vi "Create New Assert.vi"(6 "Variant in":variant, 7 "Shift Pressed?":bool, 8 "error in (no error)":errorcluster, 10 "QD Combo Box Ref":refnum<vi>, 11 "QD Launch VI Ref":refnum<vi>) -> (0 "error out":errorcluster, 4 "Variant out":variant)   [LabVIEW 2016]
doc: "Allows the user to define and insert a new assert statement onto a wire - supports I32, Double, String and Boolean data types currently\n\nDefault Shortcut - S"
panel:
  in  "Undo Name":string="Quick Drop Keyboard Shortcut"
  # "Do not change the connector pane of this VI.\n\nSee the block diagram for directions on how to use this template."
  # "Specify the name of the Undo transaction"
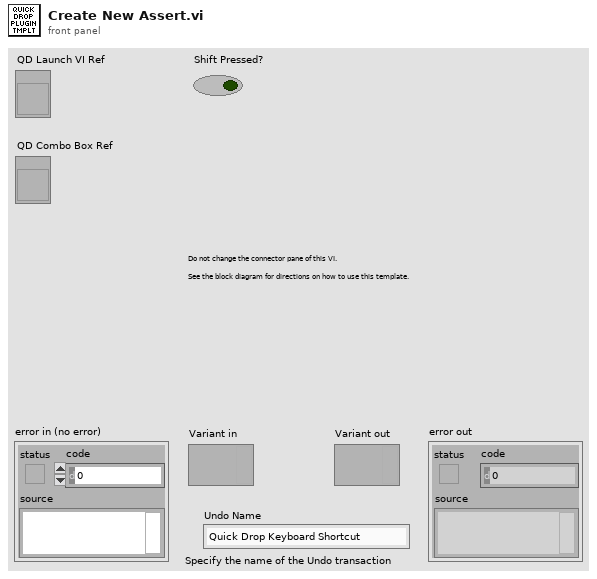
[diagram p1: front panel]
types:
  T1 = typedef "NI_Data Type.lvlib/Data Type.ctl" = enum8{"Invalid Type", "Void", "I8", "I16", "I32", "I64", "U8", "U16", "U32", "U64", "Single Float", "Double Float", "Extended Float", "Single Complex", "Double Complex", "Extended Complex", "Enum U8", "Enum U16", "Enum U32", "Enum U64", "Single Float With Unit", "Double Float With Unit", "Extended Float With Unit", "Single Complex with Unit", "Double Complex with Unit", "Extended Complex with Unit", "Boolean", "String", "Path", "Picture", "Tag", "Array", "Cluster", "Variant", "LV Variant", "Waveform", "Timestamp", "Digital Waveform", "Digital Data", "ExpressData", "Refnum", "External Data", "VI", "Poly VI", "LabVIEW Class Instance", "Fixed Point"}
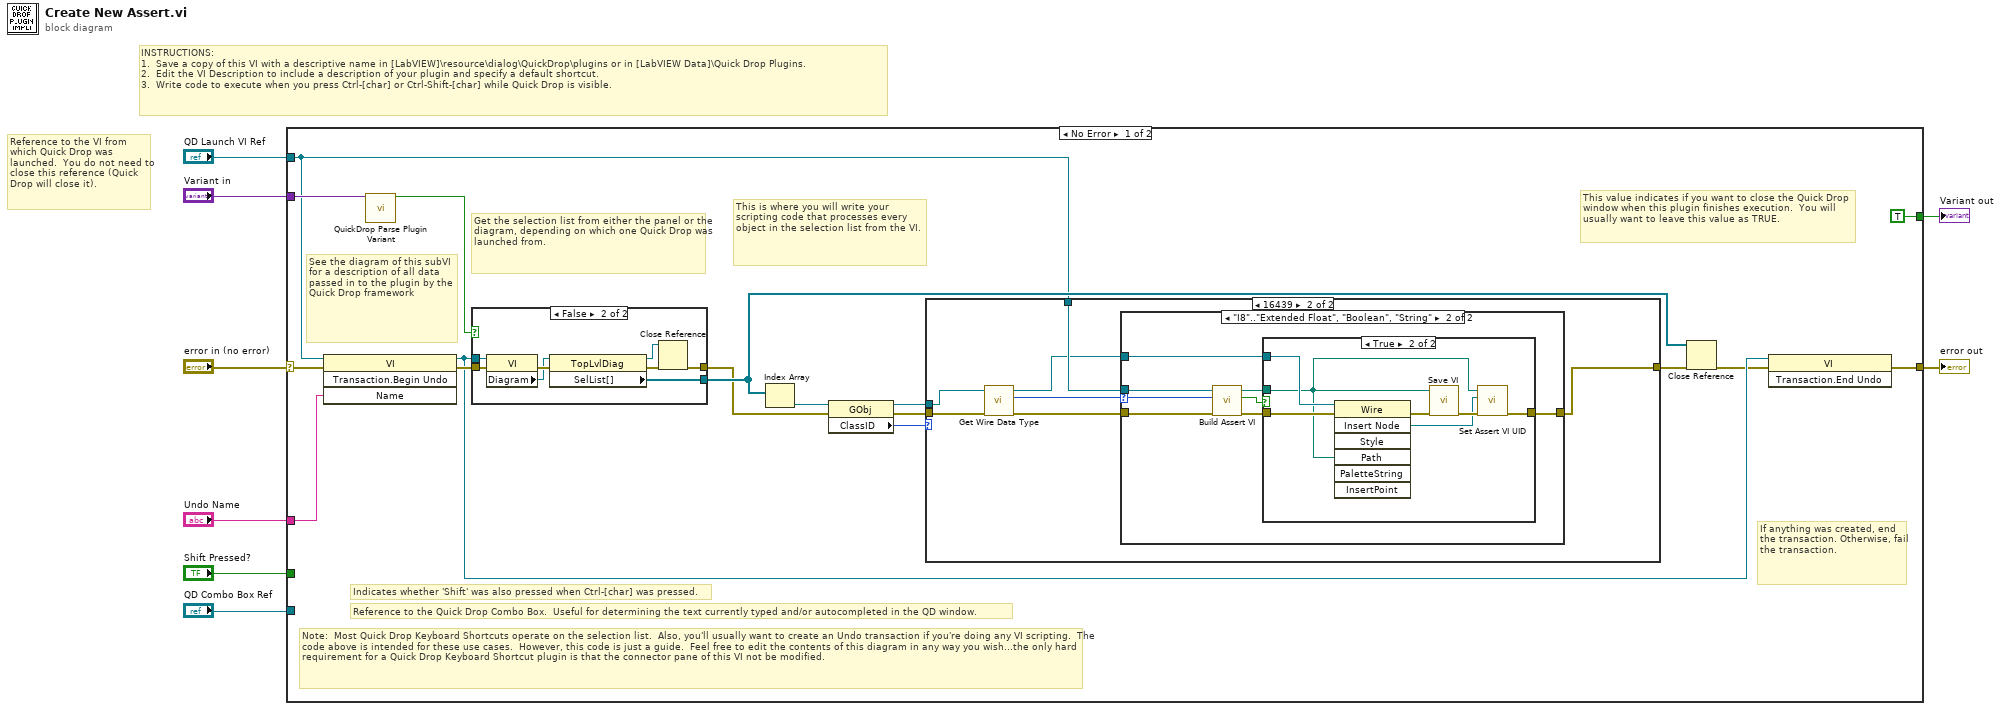
[diagram p0: block diagram]
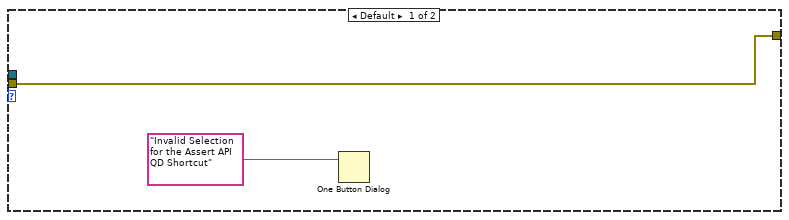
[diagram p2: hidden frame]
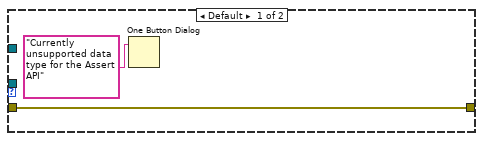
[diagram p3: hidden frame]
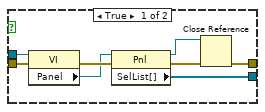
[diagram p5: hidden frame]
diagram:
  # "Reference to the VI from which Quick Drop was launched.  You do not need to close this reference (Quick Drop will close it)."
  # "INSTRUCTIONS:\n1.  Save a copy of this VI with a descriptive name in [LabVIEW]\\resource\\dialog\\QuickDrop\\plugins or in [LabVIEW Data]\\Quick Drop Plugins.\n2.  Edit the VI Description to include a description of your plugin and specify a default shortcut. \n3.  Write code to execute when you press Ctrl-[char] or Ctrl-Shift-[char] while Quick Drop is visible."
  n1 = case shown="No Error" "error in (no error)" {
    selector: "error in (no error)" -> [w24 w69]
    tunnel: [w19 w69] -> w7
    tunnel: "QD Launch VI Ref" -> [w9 _]
    tunnel: "Shift Pressed?" -> [_ _]
    tunnel: "QD Combo Box Ref" -> [_ _]
    tunnel: "Variant in" -> [w25 _]
    tunnel: "Undo Name" -> [w23 _]
    tunnel: [TRUE _] -> w1
    frame No Error {
      # "This is where you will write your scripting code that processes every object in the selection list from the VI."
      # "Note:  Most Quick Drop Keyboard Shortcuts operate on the selection list.  Also, you'll usually want to create an Undo transaction if you're doing any VI scripting.  The code above is intended for these use cases.  However, this code is just a guide.  Feel free to edit the contents of this diagram in any way you wish...the only hard requirement for a Quick Drop Keyboard Shortcut plugin is that the connector pane of this VI not be modified."
      # "Get the selection list from either the panel or the diagram, depending on which one Quick Drop was launched from."
      # "If anything was created, end the transaction. Otherwise, fail the transaction."
      # "This value indicates if you want to close the Quick Drop window when this plugin finishes execution.  You will usually want to leave this value as TRUE."
      # "See the diagram of this subVI for a description of all data passed in to the plugin by the Quick Drop framework"
      # "Reference to the Quick Drop Combo Box.  Useful for determining the text currently typed and/or autocompleted in the QD window."
      # "Indicates whether 'Shift' was also pressed when Ctrl-[char] was pressed."
      n2 = invoke class="VI" method="Transaction.Begin Undo"(reference=w9, error in=w24, "Name"=w23) -> (reference out=w18:refnum<vi>, error out=w20:errorcluster)  [unwired: 1 in, 2 out]
      n3 = call <vilib>:"QuickDrop Parse Plugin Variant.vi"("QDKS Variant in"=w25) -> ("QD Launch VI Panel?"=w21:bool)  [unwired: 12 in, 2 out]
      n4 = case shown="False" w21 {
        tunnel: w20 -> [w60 w68]
        tunnel: w18 -> [w59 w67]
        tunnel: [w54 w62] -> w14
        tunnel: [w53 w61] -> w16
        frame True {
          n5 = property class="VI"(reference=w59, error in=w60) -> (error out=w58:errorcluster, "Panel"=w57:refnum<vi>)  [unwired: 1 out]
          n6 = property class="Pnl"(reference=w57, error in=w58) -> (reference out=w55:refnum<vi>, error out=w56:errorcluster, "SelList[]"=w53:refnum<vi>[])
          n7 = Close Reference(reference=w55, error in (no error)=w56) -> (error out=w54:errorcluster)
        }
        frame False {
          n8 = property class="VI"(reference=w67, error in=w68) -> (error out=w66:errorcluster, "Diagram"=w65:refnum<vi>)  [unwired: 1 out]
          n9 = property class="TopLvlDiag"(reference=w65, error in=w66) -> (reference out=w63:refnum<vi>, error out=w64:errorcluster, "SelList[]"=w61:refnum<vi>[])
          n10 = Close Reference(reference=w63, error in (no error)=w64) -> (error out=w62:errorcluster)
        }
      }
      n11 = Index Array(array=w16) -> (element=w15:refnum<vi>)  [unwired: 1 in]
      n12 = property class="GObj"(reference=w15, error in=w14) -> (reference out=w11:refnum<vi>, error out=w12:errorcluster, "ClassID"=w13:u32)
      n13 = case shown="16439" w13 {
        tunnel: w12 -> [w26 w34]
        tunnel: w11 -> [_ w30]
        tunnel: [w26 w32] -> w10
        tunnel: w9 -> [_ w31]
        frame Default {
          n14 = One Button Dialog(message="Invalid Selection for the Assert API QD Shortcut") -> ()  [unwired: 1 in, 1 out]
        }
        frame 16439 {
          n15 = call "Get Wire Data Type.vi"("error in (no error)"=w34, "Wire ref in"=w30) -> ("error out"=w33:errorcluster, "Type"=w28:T1, "Wire ref out"=w29:refnum<vi>)  [unwired: 7 in]
          n16 = case shown="\"I8\"..\"Extended Float\", \"Boolean\", \"String\"" w28 {
            selector: w28 -> [_ w42]
            tunnel: w33 -> [w36 w44]
            tunnel: [w36 w40] -> w32
            tunnel: w31 -> [_ w43]
            tunnel: w29 -> [_ w39]
            frame Default {
              n17 = One Button Dialog(message="Currently unsupported data type for the Assert API") -> ()  [unwired: 1 in, 1 out]
            }
            frame "I8".."Extended Float", "Boolean", "String" {
              n18 = call "Build Assert VI.vi"("error in (no error)"=w44, "Type"=w42, "VI Refnum"=w43) -> ("error out"=w41:errorcluster, "Add Object"=w37:bool, "appended path"=w38:path)  [unwired: 6 in]
              n19 = case shown="True" w37 {
                tunnel: w41 -> [w45 w52]
                tunnel: [w45 w48] -> w40
                tunnel: w39 -> [_ w50]
                tunnel: w38 -> [_ w46]
                frame False {
                }
                frame True {
                  n20 = invoke class="Wire" method="Insert Node"(reference=w50, error in=w52, "Path"=w46) -> (error out=w51:errorcluster, "Insert Node"=w47:refnum<vi>)  [unwired: 4 in, 5 out]
                  n21 = call "Save VI.vi"("error in (no error)"=w51, "Assert VI Path"=w46) -> ("error out"=w49:errorcluster)  [unwired: 9 in]
                  n22 = call "Set Assert VI UID.vi"("error in (no error)"=w49, "GObj Refnum"=w47, "Assert VI Path"=w46) -> ("error out"=w48:errorcluster)  [unwired: 8 in]
                }
              }
            }
          }
        }
      }
      n23 = Close Reference(reference=w16, error in (no error)=w10) -> (error out=w17:errorcluster)
      n24 = invoke class="VI" method="Transaction.End Undo"(reference=w18, error in=w17) -> (error out=w19:errorcluster)  [unwired: 1 in, 2 out]
    }
    frame Error {
    }
  }
  "error out" <- w7
  "Variant out" <- w1
